vi "Get Total Number of Points.vi"(8 "error in":errorcluster, 11 "eye scan in":refnum<class "niHighSpeedSerial Eye Scan v1 Host.lvclass">) -> (0 "error out":errorcluster, 2 "total number of points":i32, 3 "eye scan out":refnum<class "niHighSpeedSerial Eye Scan v1 Host.lvclass">)   [LabVIEW 2014, in "niHighSpeedSerial Eye Scan v1 Host.lvclass"]
doc: "Returns the total number of points which will be measured if Eye Scan runs to completion.\n\n<B>Input Parameters</B>\n\n<B>error in</B> describes error conditions that occur before this node runs. This input provides standard 'error in' functionality.\n\n<B>eye scan in</B> Takes in a reference to your session from the previous VI.\n\n<B>Output Parameters</B>\n\n<B>error out</B> contains error information. This output provides standard 'error out' functionality.\n\n<B>total number of points</B> is the total number of points which will be measured if Eye Scan runs to completion.\n\n<B>eye scan out</B> passes a reference to your session to the next VI."
uses:
  <instrlib>/niHighSpeedSerial/Eye Scan/v1/Host/Eye Scan/niHighSpeedSerial Eye Scan v1 Host.lvclass
  <instrlib>/niHighSpeedSerial/Eye Scan/v1/Host/Eye Scan/niHighSpeedSerial Eye Scan v1 Host.lvclass/niHighSpeedSerial Eye Scan v1 Host.ctl
  <vilib>/Utility/error.llb/Error Cluster From Error Code.vi
  <vilib>/ErrorRing/Error Ring.xnode
  <instrlib>/niHighSpeedSerial/Eye Scan/v1/Host/Impl/Eye Scan Point Iterator/niHighSpeedSerial Eye Scan Point Iterator v1 Host.lvclass
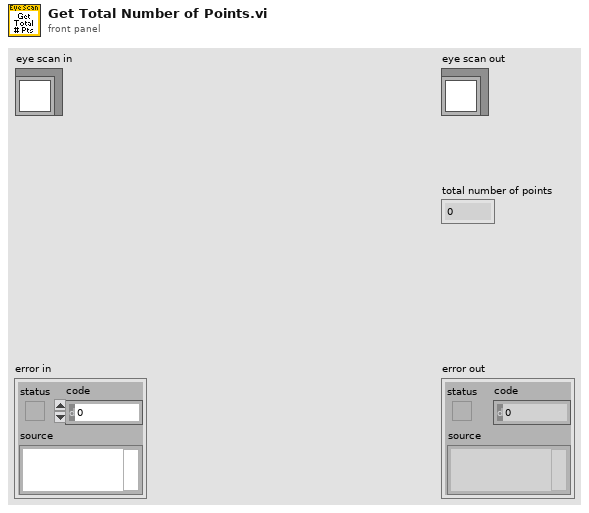
[diagram p1: front panel]
types:
  T1 = typedef "niHighSpeedSerial Eye Scan v1 Host.lvclass/Private Data.ctl" = cluster{"instruction target":refnum<class "niInstr Instruction Target v1 Host.lvclass">, "channels":T2[], "measure state":T3, "rx output divider":T4, "equalization mode":T5, "rx data width":T6, "BER floor":dbl, "number of points completed":i32, "rx output divider configured?":bool, "equalization mode configured?":bool, "rx data width configured?":bool}
  T2 = typedef "niHighSpeedSerial Eye Scan v1 Host.lvclass/Channel Data.ctl" = cluster{"instance":u8, "channel":refnum<class "niHighSpeedSerial Eye Scan Single Point v1 Host.lvclass">, "point iterator":refnum<class "niHighSpeedSerial Eye Scan Point Iterator v1 Host.lvclass">}
  T3 = typedef "niHighSpeedSerial Eye Scan v1 Host.lvclass/Measure State.ctl" = enum16{"Uninitialized", "Initialized", "Ready", "Measuring", "Finished", "Aborted"}
  T4 = typedef "niHighSpeedSerial Eye Scan Common v1 Host.lvlib/RX Output Divider.ctl" = enum16{"1", "2", "4", "8", "16"}
  T5 = typedef "niHighSpeedSerial Eye Scan Common v1 Host.lvlib/Equalization Mode.ctl" = enum16{"DFE", "LPM"}
  T6 = typedef "niHighSpeedSerial Eye Scan Common v1 Host.lvlib/Data Width.ctl" = enum16{"16 Bit", "20 Bit", "32 Bit", "40 Bit"}
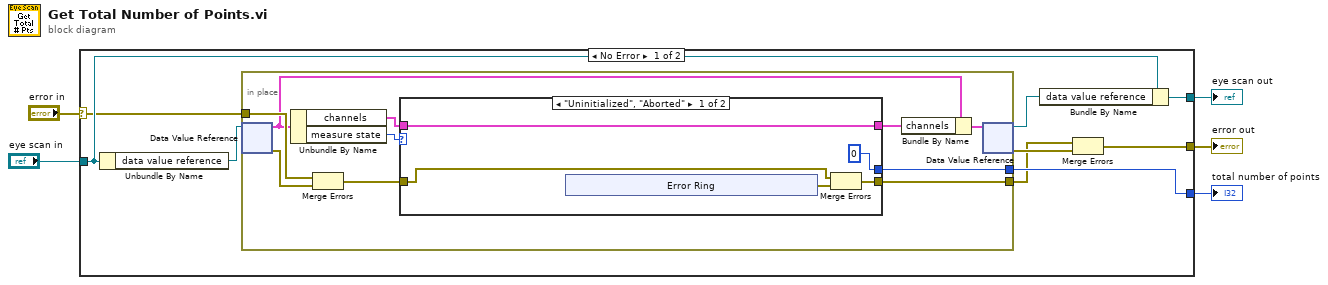
[diagram p0: block diagram]
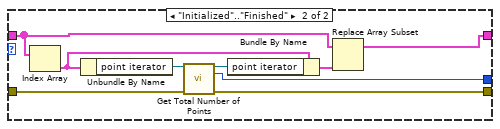
[diagram p2: hidden frame]
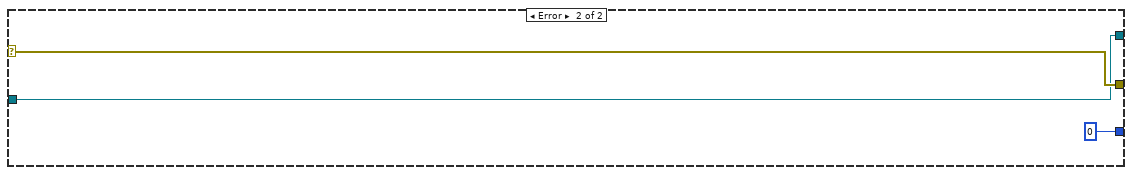
[diagram p3: hidden frame]
diagram:
  n1 = case shown="No Error" "error in" {
    selector: "error in" -> [w9 w45]
    tunnel: [w6 w45] -> w2
    tunnel: [w11 w44] -> w3
    tunnel: "eye scan in" -> [w10 w44]
    tunnel: [w14 0 ("Total Number of Points")] -> w1
    frame No Error {
      n2 = Unbundle By Name(w10) -> ("data value reference"=w13:refnum<data-value>)
      n3 = in-place {
        in-place-border: [w24] -> w14
        in-place-border: w9 -> [w23]
        in-place-border: [w20] -> w7
        n4 = in-place-dvr #1(w13) -> (w18:T1, w22:errorcluster)
        n5 = Unbundle By Name(w18) -> ("channels"=w19:T2[], "measure state"=w15:T3)
        n6 = Merge Errors(w23, w22) -> (w21:errorcluster)
        n7 = case shown="\"Uninitialized\", \"Aborted\"" w15 {
          tunnel: [0 ("total number of points") w42] -> w24
          tunnel: w21 -> [w27 w40]
          tunnel: [w26 w39] -> w20
          tunnel: w19 -> [w29 w36]
          tunnel: [w29 w34] -> w17
          frame "Uninitialized", "Aborted" {
            n8 = xnode "Error Ring"() -> ("error out"=w25:errorcluster)
            n9 = Merge Errors(w27, w25) -> (w26:errorcluster)
          }
          frame "Initialized".."Finished" {
            n10 = Index Array(array=w36) -> (element=w38:T2)  [unwired: 1 in]
            n11 = Unbundle By Name(w38) -> ("point iterator"=w41:refnum<class "niHighSpeedSerial Eye Scan Point Iterator v1 Host.lvclass">)
            n12 = call-dynamic "Get Total Number of Points.vi"("eye scan point iterator"=w41, "error in"=w40) -> ("eye scan point iterator out"=w37:refnum<class "niHighSpeedSerial Eye Scan Point Iterator v1 Host.lvclass">, "total number of points"=w42:i32, "error out"=w39:errorcluster)  [unwired: 11 in]
            n13 = Bundle By Name(cluster=w38, "point iterator"=w37) -> (w35:T2)
            n14 = Replace Array Subset(array=w36, new element=w35) -> (w34:T2[])  [unwired: 1 in]
          }
        }
        n15 = Bundle By Name(cluster=w18, "channels"=w17) -> (w16:T1)
        n16 = in-place-dvr #1(w16) -> (w12:refnum<data-value>, w8:errorcluster)
      }
      n17 = Bundle By Name(cluster=w10, "data value reference"=w12) -> (w11:refnum<class "niHighSpeedSerial Eye Scan v1 Host.lvclass">)
      n18 = Merge Errors(w7, w8) -> (w6:errorcluster)
    }
    frame Error {
    }
  }
  "error out" <- w2
  "eye scan out" <- w3
  "total number of points" <- w1
